vi "Data_base_server.vi"(0 "Raw Data Pathname":path, 1 "Results File Pathname":path, 3 "Clients time":dbl, 4 "Start time":dbl, 5 "End time":dbl, 6 "Average Meas Time (min)":dbl=100.0 format="%.1f", 7 "Channels from Client":string[][](array[string])=[["Data Base:Measurement:Type", "LDA & Cw"], ["Data Base:Position:No of Inst", "2"], ["Data Base:Position:X1", "-60"], ["Data Base:Position:X2", ""], ["Data Base:Position:Y1", "2"], ["Data Base:Position:Y2", "0.00"], ["Data Base:Position:Z1", "0.00"], ["Data Base:Position:Z2", "2.00"]], 8 "Average Sampling freq":sgl=100.0 format="%.1f", 9 "Rig Name":string) -> (14 "Channel names":string[](array[string])=["Data Base:DB:Filename", "Data Base:Start:Date", "Data Base:Start:Time", "EnFlo Tun:Job: Name", "EnFlo Tun:User: Name", "Data Base:Results:Folder", "Data Base:Results:Filename", "Data Base:Measurement:Type", "Data Base:X Axis:Max", "Data Base:X Axis:Min", "Data Base:Y Axis:Max", "Data Base:Y Axis:Min", "Data Base:Z Axis:Max", "Data Base:Z Axis:Min", "Data Base:No of:Measurements", "Data Base:Av Meas:Frequency (Hz)", "Data Base:Av Meas:Time (min)", "EnFlo Tun:labstrat1:Delta T", "EnFlo Tun:Heater Temp:Average", "EnFlo Tun:Inside:Velocity", "EnFlo Tun:Vorticity: Generators", "EnFlo Tun:Barrier Wall: Height", "EnFlo Tun:Roughness: Height", "EnFlo Tun:Side Wall: Separation", "EnFlo Tun:Obstacle/:Building", "EnFlo Tun:Obstacle: Orientation", "GMU:Source: Type", "GMU:Source: Height", "GMU:Release: Orientation", "GMU:Source:Meas Q", "GMU:Source:Meas Strength", "GMU:Trace: Gas", "GMU:Carrier: Gas", "GMU:Source:Release Temp", "GMU:Suction:Meas Q"], 15 "Channel values":string[](array[string])=["1999:May_1999:G3_3 HD_00006", "13/5/99", "1:55 pm", "National Power", "Paul Hayden", "BMT", "default", "LDA, Cw", "100.00", "-60.00", "2.00", "0.00", "0.00", "0.00", "10", "100.00", "100.00", "1.42", "26.63", "1.54", "\"7 quarter elipticals, 1 metre tall\"", "150mm", "20mm", "No sidewalls installed", "National Power Building", "30 deg", "D=17.5mm", "150 mm", "Vertical", "", "", "Ethane", "48% N2 in He", "", ""], 17 "spreadsheet string":string)   [LabVIEW 2022 SP3]
doc: "This is an example of using features of the VI Server as a client. It shows how you might browse from one or more applications that may be exporting data from one or more data stations. \n\nThe example shows how to query a server for its list of exported VIs, how to get references to the VIs, and how call them with the Call By Reference function."
uses:
  ADAM_Global.vi
  Sub VI's/Exp conditions/EnFlo_Tun_Setup_global.vi
  Anemometry/Anemometry Sub Vis/Globals/Constants_global.vi
panel:
  out "Output Array":string[][](array[string])
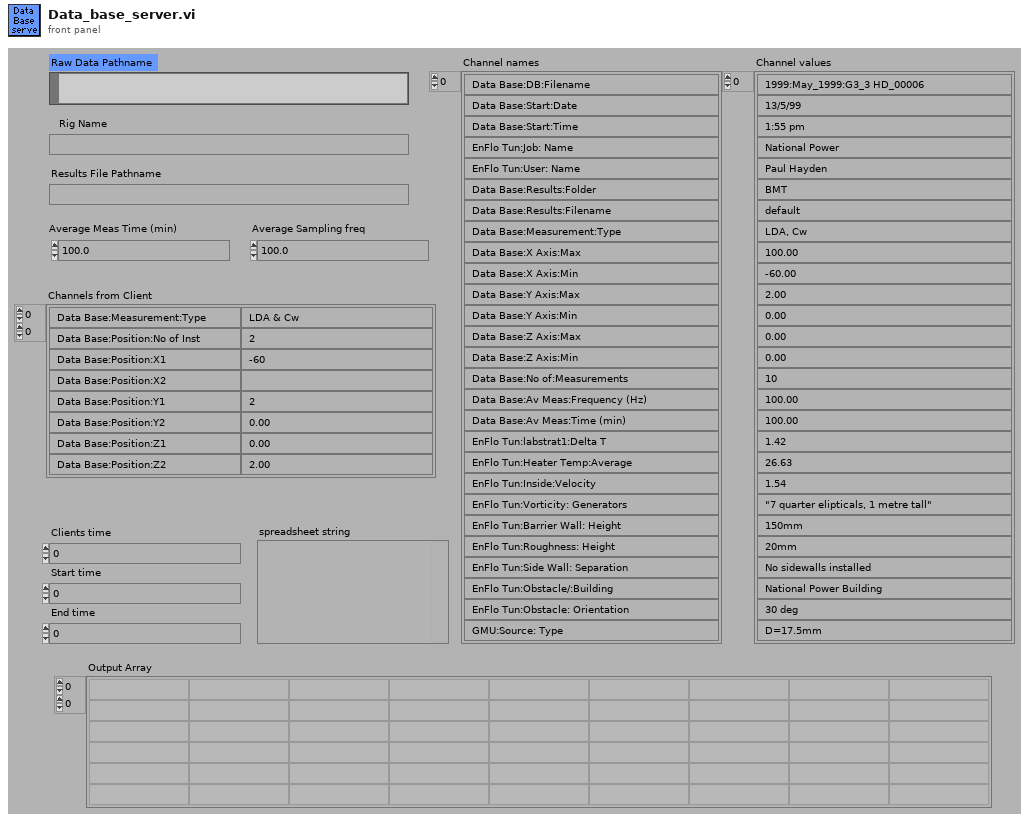
[diagram p1: front panel]
types:
  T1 = typedef "Ch_description_ADAM.ctl" = cluster{"Ch Name":string, "Type":T2, "Function":T3, "Ch State":T4, "Calibration type":T5, "A":dbl, "B":dbl, "C":dbl, "D":dbl, "Comments":string, "Address":T6, "String":string, "Duty":u16}
  T2 = typedef "Module_type_ADAM.ctl" = string
  T3 = typedef "Function_ADAM.ctl" = enum16{"Analogue Input", "Digital Input", "Event counter", "Event rate", "Analogue Output", "Digital Output", "Relay Output"}
  T4 = typedef "Channel_State.ctl" = enum16{"On", "Off", "Always On", "Always Off"}
  T5 = typedef "Calib_type_ADAM.ctl" = string
  T6 = typedef "Address.ctl" = cluster{"Main":i32, "Ch.":i32, "Sub":i32, "Port Name":string}
  T7 = cluster{"second":i32, "minute":i32, "hour":i32, "day of month":i32, "month":i32, "year":i32, "day of week":i32, "day of year":i32, "is DST":i32}
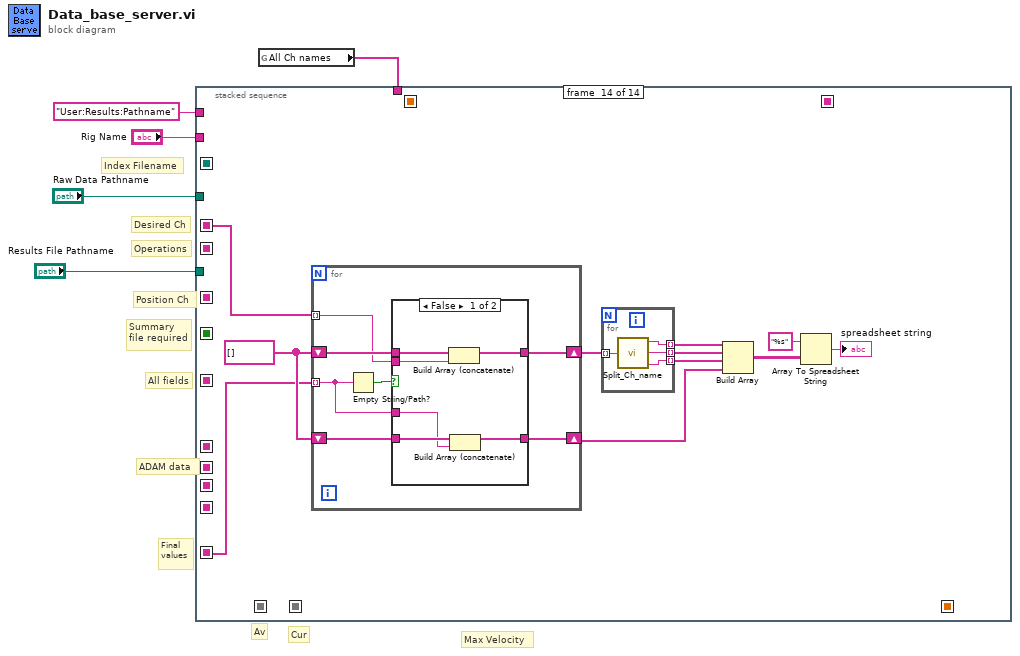
[diagram p0: block diagram]
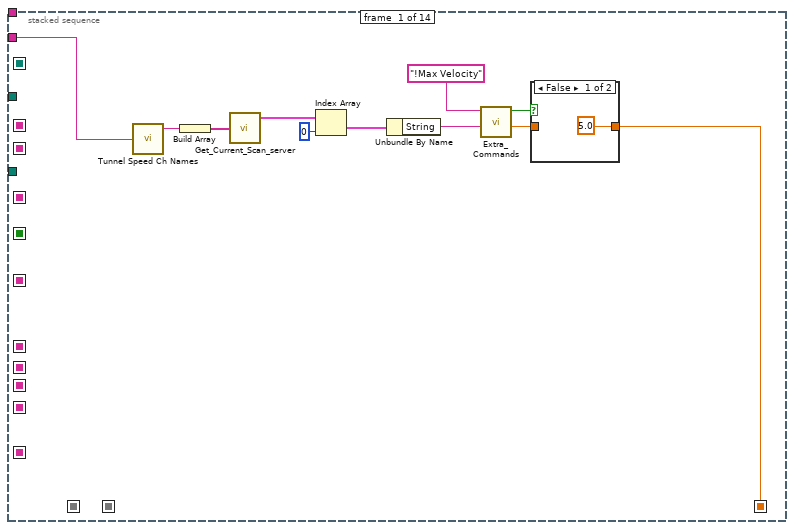
[diagram p2: hidden frame]
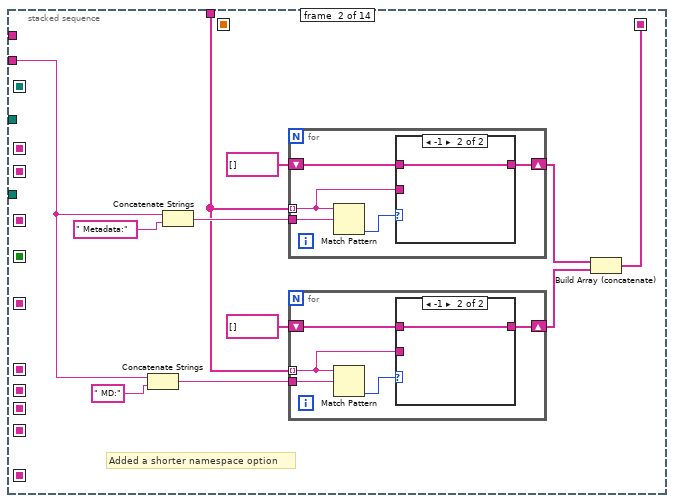
[diagram p4: hidden frame]
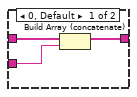
[diagram p5: hidden frame]
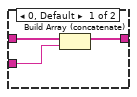
[diagram p6: hidden frame]
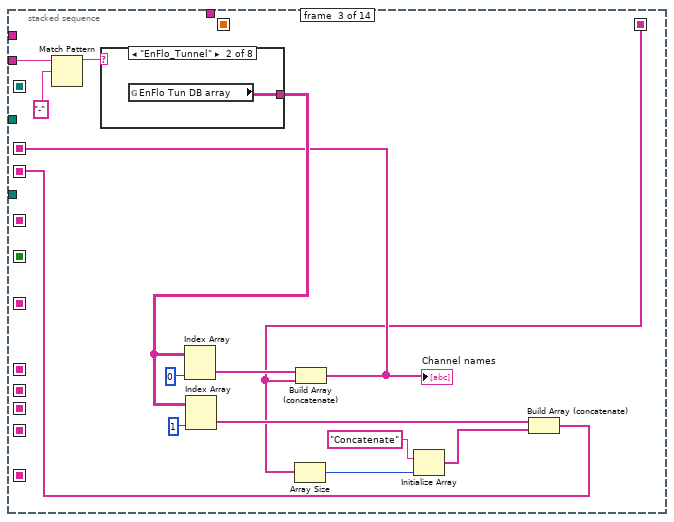
[diagram p7: hidden frame]
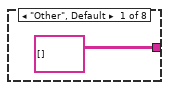
[diagram p8: hidden frame]
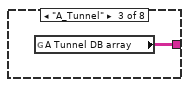
[diagram p9: hidden frame]
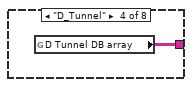
[diagram p10: hidden frame]
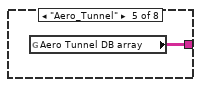
[diagram p11: hidden frame]
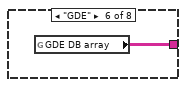
[diagram p12: hidden frame]
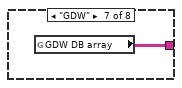
[diagram p13: hidden frame]
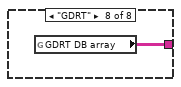
[diagram p14: hidden frame]
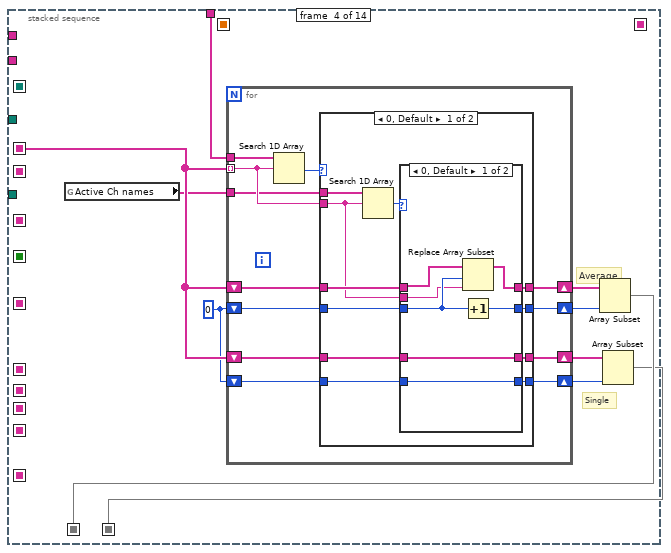
[diagram p15: hidden frame]
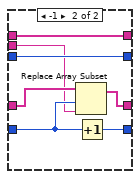
[diagram p16: hidden frame]
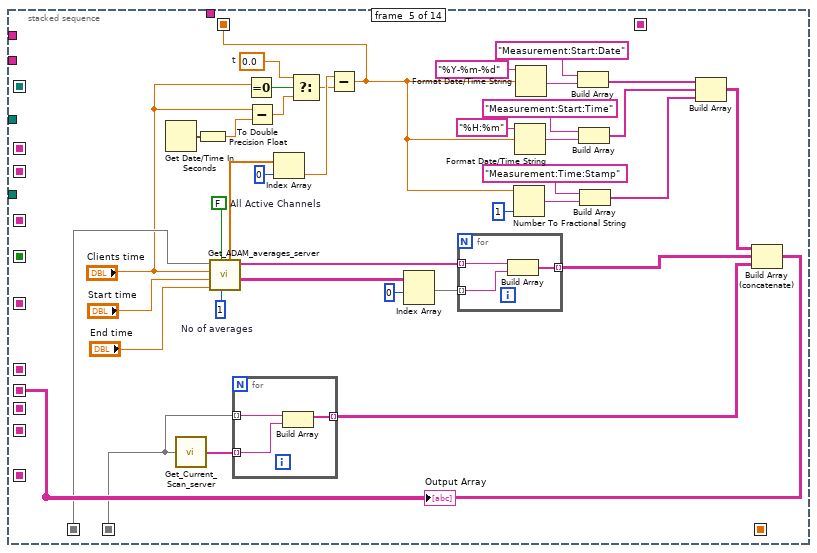
[diagram p18: hidden frame]
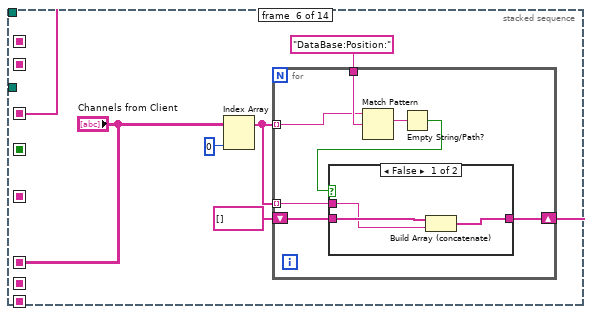
[diagram p19: hidden frame]
diagram:
  # "Max Velocity"
  # "Cur"
  # "Av"
  # "Index Filename"
  # "Desired Ch"
  # "Operations"
  # "Final\nvalues"
  # "Summary\nfile required"
  # "Position Ch"
  # "All fields"
  # "ADAM data"
  n1 = global read "ADAM_Global.vi" "All Ch names"() -> (w3:string[])
  n2 = stacked-sequence {
    seq-local: [_ _ w57 _ _ _ _ _ _ _ _ _ _ _] -> [_ _ _ w79 _ _ _ _ _ w218 _ _ w353 w363]
    seq-local: [_ _ _ _ w149 _ _ _ _ _ _ _ _ _] -> [_ _ _ _ _ _ _ _ w212 _ _ _ _ _]
    seq-local: [_ _ _ _ _ _ w199 _ _ _ _ _ _ _] -> [_ _ _ _ _ _ _ _ w211 _ _ _ _ _]
    seq-local: [_ _ _ _ _ _ _ _ w208 _ _ _ _ _] -> [_ _ _ _ _ _ _ _ _ w216 w318 _ _ _]
    seq-local: [_ _ _ _ _ _ _ w203 _ _ _ _ _ _] -> [_ _ _ _ _ _ _ _ w210 _ _ _ _ _]
    seq-local: [_ _ _ _ _ _ _ _ _ w220 _ _ _ _] -> [_ _ _ _ _ _ _ _ _ _ w324 _ w354 w362]
    seq-local: [_ _ _ _ _ w166 _ _ _ _ _ _ _ _] -> [_ _ _ _ _ _ _ w206 _ w217 _ _ _ _]
    seq-local: [_ _ _ _ _ "Channels from Client" _ _ _ _ _ _ _ _] -> [_ _ _ _ _ _ _ _ w209 w213 _ _ _ _]
    seq-local: [_ _ _ _ _ _ _ w204 _ _ _ _ _ _] -> [_ _ _ _ _ _ _ _ _ w219 _ _ _ _]
    seq-local: [_ _ w51 _ _ _ _ _ _ _ _ _ _ _] -> [_ _ _ _ _ _ _ _ _ w215 _ _ _ _]
    seq-local: [_ _ _ _ w123 _ _ _ _ _ _ _ _ _] -> [_ _ _ _ _ _ _ _ _ _ _ _ _ _]
    seq-local: [_ _ _ _ _ _ _ _ _ _ _ w341 _ _] -> [_ _ _ _ _ _ _ _ _ _ _ _ w351 _]
    seq-local: [_ _ _ w72 _ _ _ _ _ _ _ _ _ _] -> [_ _ _ _ w141 _ _ _ _ _ _ _ _ _]
    seq-local: [_ _ _ w71 _ _ _ _ _ _ _ _ _ _] -> [_ _ _ _ w140 _ _ _ _ _ _ _ _ _]
    seq-local: [_ w19 _ _ _ _ _ _ _ _ _ _ _ _] -> [_ _ w54 _ _ _ _ _ _ _ _ _ _ _]
    seq-local: [w7 _ _ _ _ _ _ _ _ _ _ _ _ _] -> [_ _ _ _ _ _ _ _ _ _ w311 _ _ _]
    tunnel: "User:Results:Pathname" -> [_ _ _ _ _ _ w187 _ _ _ _ _ w355 _]
    tunnel: "Results File Pathname" -> [_ _ _ _ _ _ w184 _ _ w214 _ _ _ _]
    tunnel: "Rig Name" -> [w16 w23 w50 _ _ _ _ _ _ _ w310 w348 _ _]
    tunnel: w3 -> [_ w24 _ w70 _ _ _ _ _ _ _ _ _ _]
    tunnel: "Raw Data Pathname" -> [_ _ _ _ _ _ _ w202 _ _ _ _ _ _]
    frame #0 {
      n3 = call "Tunnel Speed Ch Names.vi"("Rig Name"=w16) -> ("Dem Velocity"=w15:string)  [unwired: 2 in, 2 out]
      n4 = Build Array(w15) -> (w14:string[])
      n5 = call "Get_Current_Scan_server.vi"("Desired Channels"=w14) -> ("Ch Description Array"=w10:T1[])  [unwired: 2 out]
      n6 = Index Array(array=w10, index=0 ("Index")) -> (element=w13:T1)
      n7 = Unbundle By Name(w13) -> ("String"=w12:string)
      n8 = call "Extra_Commands.vi"("String to Search"=w12, "Command"="!Max Velocity") -> ("Numeric Value"=w6:dbl, "Command Found"=w8:bool)  [unwired: 1 in, 3 out]
      n9 = case shown="False" w8 {
        tunnel: [5.0 ("Max Velocity") w18] -> w7
        tunnel: w6 -> [_ w18]
        frame False {
        }
        frame True {
        }
      }
    }
    frame #1 {
      # "Added a shorter namespace option"
      n10 = Concatenate Strings(w23, " MD:" ("string")) -> (w25:string)
      n11 = Concatenate Strings(w23, " Metadata:") -> (w28:string)
      n12 = for {
        tunnel: w28 -> [w40]
        shift-right: [w41] -> w20
        shift-left: string[] [] -> [w42]
        tunnel: w24 -> [w39] mode=indexing
        n13 = Match Pattern(string=w39, regular expression=w40) -> (offset past match=w43:i32)  [unwired: 4 out]
        n14 = case shown="-1" w43 {
          tunnel: w42 -> [w46 w47]
          tunnel: [w44 w47] -> w41
          tunnel: w39 -> [w45 _]
          frame 0, Default {
            n15 = Build Array (concatenate)(w46, w45) -> (w44:string[])
          }
          frame -1 {
          }
        }
      }
      n16 = for {
        tunnel: w25 -> [w31]
        shift-right: [w32] -> w21
        shift-left: string[] [] -> [w33]
        tunnel: w24 -> [w30] mode=indexing
        n17 = Match Pattern(string=w30, regular expression=w31) -> (offset past match=w34:i32)  [unwired: 4 out]
        n18 = case shown="-1" w34 {
          tunnel: w33 -> [w37 w38]
          tunnel: [w35 w38] -> w32
          tunnel: w30 -> [w36 _]
          frame 0, Default {
            n19 = Build Array (concatenate)(w37, w36) -> (w35:string[])
          }
          frame -1 {
          }
        }
      }
      n20 = Build Array (concatenate)(w20, w21) -> (w19:string[])
    }
    frame #2 {
      n21 = Match Pattern(string=w50, regular expression="-") -> (before substring=w48:string)  [unwired: 1 in, 3 out]
      n22 = case shown="\"EnFlo_Tunnel\"" w48 {
        tunnel: [string[][] [] ("EnFlo Tun DB array") w63 w64 w65 w66 w67 w68 w69] -> w59
        frame "Other", Default {
        }
        frame "EnFlo_Tunnel" {
          n23 = global read "EnFlo_Tun_Setup_global.vi" "EnFlo Tun DB array"() -> (w63:string[][])
        }
        frame "A_Tunnel" {
          n24 = global read "EnFlo_Tun_Setup_global.vi" "A Tunnel DB array"() -> (w64:string[][])
        }
        frame "D_Tunnel" {
          n25 = global read "EnFlo_Tun_Setup_global.vi" "D Tunnel DB array"() -> (w65:string[][])
        }
        frame "Aero_Tunnel" {
          n26 = global read "EnFlo_Tun_Setup_global.vi" "Aero Tunnel DB array"() -> (w66:string[][])
        }
        frame "GDE" {
          n27 = global read "EnFlo_Tun_Setup_global.vi" "GDE DB array"() -> (w67:string[][])
        }
        frame "GDW" {
          n28 = global read "EnFlo_Tun_Setup_global.vi" "GDW DB array"() -> (w68:string[][])
        }
        frame "GDRT" {
          n29 = global read "EnFlo_Tun_Setup_global.vi" "GDRT DB array"() -> (w69:string[][])
        }
      }
      n30 = Index Array(array=w59, index (col)=0) -> (element=w58:string[])  [unwired: 1 in]
      n31 = Index Array(array=w59, index (col)=1) -> (element=w56:string[])  [unwired: 1 in]
      n32 = Array Size(array=w54) -> (size(s)=w55:i32)
      n33 = Build Array (concatenate)(w58, w54) -> (w57:string[])
      "Channel names" <- w57
      n34 = Initialize Array("Concatenate", w55) -> (w52:string[])
      n35 = Build Array (concatenate)(w56, w52) -> (w51:string[])
    }
    frame #3 {
      w77 = 0
      # "Single"
      # "Average"
      n36 = global read "ADAM_Global.vi" "Active Ch names"() -> (w78:string[])
      n37 = for {
        tunnel: w79 -> [w85] mode=indexing
        tunnel: w70 -> [w91]
        shift-right: [w89] -> w76
        shift-left: w79 -> [w88]
        shift-right: [w87] -> w74
        shift-left: w79 -> [w86]
        tunnel: w78 -> [w84]
        shift-right: [w80] -> w75
        shift-left: w77 -> [w81]
        shift-right: [w82] -> w73
        shift-left: w77 -> [w83]
        n38 = Search 1D Array(1D array=w91, element=w85) -> (index of element=w90:i32)  [unwired: 1 out]
        n39 = case shown="0, Default" w90 {
          tunnel: [w93 w120] -> w89
          tunnel: w88 -> [w94 w120]
          tunnel: [w99 w119] -> w87
          tunnel: w86 -> [w100 w119]
          tunnel: w85 -> [w92 _]
          tunnel: w84 -> [w102 _]
          tunnel: w83 -> [w98 w117]
          tunnel: [w97 w117] -> w82
          tunnel: w81 -> [w96 w118]
          tunnel: [w95 w118] -> w80
          frame 0, Default {
            n40 = Search 1D Array(1D array=w102, element=w92) -> (index of element=w101:i32)  [unwired: 1 out]
            n41 = case shown="0, Default" w101 {
              tunnel: w100 -> [w105 w116]
              tunnel: [w105 w115] -> w99
              tunnel: w98 -> [w104 w114]
              tunnel: [w104 w113] -> w97
              tunnel: w96 -> [w109 w112]
              tunnel: [w106 w112] -> w95
              tunnel: w94 -> [w108 w111]
              tunnel: [w107 w111] -> w93
              tunnel: w92 -> [w103 w110]
              frame 0, Default {
                n42 = Replace Array Subset(array=w108, new element=w103, index=w109) -> (w107:string[])
                n43 = Increment(x=w109) -> (x+1=w106:i32)
              }
              frame -1 {
                n44 = Replace Array Subset(array=w116, new element=w110, index=w114) -> (w115:string[])
                n45 = Increment(x=w114) -> (x+1=w113:i32)
              }
            }
          }
          frame -1 {
          }
        }
      }
      n46 = Array Subset(array=w76, length=w75) -> (w72:string[])  [unwired: 1 in]
      n47 = Array Subset(array=w74, length=w73) -> (w71:string[])  [unwired: 1 in]
    }
    frame #4 {
      w134 = 0.0  # t
      w142 = FALSE  # All Active Channels
      w158 = 1  # No of averages
      n48 = Get Date/Time In Seconds() -> (seconds since 1Jan1904=w130:timestamp)
      n49 = call "Get_Current_Scan_server.vi"("Desired Channels"=w140) -> ("String values"=w139:string[])  [unwired: 2 out]
      n50 = To Double Precision Float(number=w130) -> (double precision float=w137:dbl)
      n51 = call "Get_ADAM_averages_server.vi"("No of averages"=w158, "All Active Channels"=w142, "End time"="End time", "Start time"="Start time", "Clients time"="Clients time", "ADAM Ch Names"=w141) -> ("Values"=w145:string[][], "Titles"=w148:string[], "Times"=w156:dbl[])  [unwired: 2 out]
      n52 = for {
        tunnel: w139 -> [w161] mode=indexing
        tunnel: [w160] -> w138 mode=indexing
        tunnel: w140 -> [w159] mode=indexing
        n53 = Build Array(w159, w161) -> (w160:string[])
      }
      n54 = Equal To 0?(x="Clients time") -> (x = 0?=w135:bool)
      n55 = Subtract(x="Clients time", y=w137) -> (x-y=w136:dbl)
      n56 = Index Array(array=w156, index=0) -> (element=w132:dbl)
      n57 = Select(t=w134, s=w135, f=w136) -> (s? t:f=w131:dbl)
      n58 = Subtract(x=w132, y=w131) -> (x-y=w123:dbl)
      n59 = Index Array(array=w145, index (row)=0) -> (element=w147:string[])  [unwired: 1 in]
      n60 = for {
        tunnel: w148 -> [w164] mode=indexing
        tunnel: w147 -> [w163] mode=indexing
        tunnel: [w162] -> w150 mode=indexing
        n61 = Build Array(w164, w163) -> (w162:string[])
      }
      n62 = Number To Fractional String(number=w123, precision (6)=i16 1) -> (F-format string=w122:string)  [unwired: 2 in]
      n63 = Format Date/Time String(time format string (%c)="%H:%m", seconds (now)=w123) -> (date/time string=w126:string)  [unwired: 1 in]
      n64 = Format Date/Time String(time format string (%c)="%Y-%m-%d", seconds (now)=w123) -> (date/time string=w128:string)  [unwired: 1 in]
      n65 = Build Array("Measurement:Start:Date", w128) -> (w153:string[])
      n66 = Build Array("Measurement:Start:Time", w126) -> (w152:string[])
      n67 = Build Array("Measurement:Time:Stamp", w122) -> (w124:string[])
      n68 = Build Array(w153, w152, w124) -> (w151:string[][])
      n69 = Build Array (concatenate)(w151, w150, w138) -> (w149:string[][])
      "Output Array" <- w149
    }
    frame #5 {
      n70 = Index Array(array="Channels from Client", index (col)=0) -> (element=w168:string[])  [unwired: 1 in]
      n71 = for {
        tunnel: "DataBase:Position:" ("String to match") -> [w177]
        tunnel: w168 -> [w176] mode=indexing
        shift-right: [w171] -> w166
        shift-left: string[] [] -> [w172]
        tunnel: w168 -> [w173] mode=indexing
        n72 = Match Pattern(string=w176, regular expression=w177) -> (match substring=w175:string)  [unwired: 4 out]
        n73 = Empty String/Path?(string/path=w175) -> (empty?=w174:bool)
        n74 = case shown="False" w174 {
          tunnel: w173 -> [w178 _]
          tunnel: w172 -> [w180 w181]
          tunnel: [w179 w181] -> w171
          frame False {
            n75 = Build Array (concatenate)(w180, w178) -> (w179:string[])
          }
          frame True {
          }
        }
      }
    }
    frame #6 {
      n76 = Path To String(path=w184) -> (string=w186:string)
      n77 = Strip Path(path=w184) -> (name=w183:string)  [unwired: 1 out]
      n78 = Number To Fractional String(number="Average Meas Time (min)", precision (6)=i16 2) -> (F-format string=w196:string)  [unwired: 2 out]
      n79 = Number To Fractional String(number="Average Sampling freq", precision (6)=i16 2) -> (F-format string=w194:string)  [unwired: 2 out]
      n80 = Build Array("DataBase:Av Meas:Time (min)", w196) -> (w190:string[])
      n81 = Build Array("DataBase:Av Meas:Frequency (Hz)", w194) -> (w189:string[])
      n82 = Build Array("User:Results:Filename", w183) -> (w182:string[])
      n83 = Build Array(w187, w186) -> (w188:string[])
      n84 = Build Array(w188, w182, w190, w189) -> (w199:string[][])
    }
    frame #7 {
      n85 = Array Size(array=w206) -> (size(s)=w205:i32)
      n86 = Not Equal To 0?(x=w205) -> (x != 0?=w204:bool)
      n87 = Strip Path(path=w202) -> (stripped path=w201:path)  [unwired: 1 out]
      n88 = call "Path_2_String.vi"("Real Path"=w201) -> ("Path String"=w200:string)
      n89 = Build Array("DataBase:Raw_Data:Folder", w200) -> (w203:string[])
    }
    frame #8 {
      n90 = Build Array (concatenate)(w209, w212, w211, w210) -> (w208:string[][])
    }
    frame #9 {
      n91 = case shown="True" w219 {
        tunnel: [w222 w234] -> w220
        tunnel: w218 -> [w223 w233]
        tunnel: w217 -> [_ w232]
        tunnel: w216 -> [w224 w231]
        tunnel: w215 -> [_ w230]
        tunnel: w214 -> [_ w229]
        tunnel: w213 -> [_ w228]
        frame False {
          n92 = Index Array(array=w224, index (col)=1) -> (element=w225:string[])  [unwired: 1 in]
          n93 = Index Array(array=w224, index (col)=0) -> (element=w221:string[])  [unwired: 1 in]
          n94 = call "Merge_row_values.vi"("Present Row values"=w225, "Present Channels"=w221, "Desired Channels"=w223) -> ("Desired Row values"=w222:string[])  [unwired: 1 out]
        }
        frame True {
          # "Exists?"
          # "Ch names"
          # "Values"
          n95 = stacked-sequence {
            seq-local: [_ _ w265 _ _] -> [_ _ _ w281 w303]
            seq-local: [_ _ w261 _ _] -> [_ _ _ w285 w305]
            seq-local: [w242 _ _ _ _] -> [_ w248 w263 _ w306]
            seq-local: [_ w245 _ _ _] -> [_ _ w257 _ w304]
            seq-local: [_ _ w258 _ _] -> [_ _ _ _ w302]
            tunnel: [_ _ _ w286 _] -> w234
            tunnel: w233 -> [_ _ w264 w283 _]
            tunnel: w232 -> [_ _ w271 _ _]
            tunnel: w231 -> [_ _ w267 _ _]
            tunnel: w230 -> [_ _ _ w284 _]
            tunnel: w229 -> [w243 _ _ _ _]
            tunnel: w228 -> [_ w251 _ _ _]
            frame #0 {
              n96 = Strip Path(path=w243) -> (name=w236:string)  [unwired: 1 out]
              n97 = call "Add_filename_suffix.vi"("Filename"=w236) -> ("Base name"=w235:string)  [unwired: 1 in, 3 out]
              n98 = global read "Constants_global.vi" "Data Folder Local"() -> (w241:path)
              n99 = Concatenate Strings(w235, "_Sum.xls" ("Substring")) -> (w237:string)
              n100 = Build Array("Results_Summary_files", w237) -> (w240:string[])
              n101 = call "Build_Pathname.vi"("PathElements"=w240, "PathnameIn"=w241) -> ("AppendedPath"=w238:path)
              n102 = call "Create_directory_path.vi"("Path name"=w238) -> ("Path name Out"=w242:path)  [unwired: 2 in, 1 out]
            }
            frame #1 {
              n103 = Index Array(array=w251, index (col)=0) -> (element=w255:string[])  [unwired: 1 in]
              n104 = Search 1D Array(1D array=w255, element="Does the results file already exist?") -> (index of element=w252:i32)  [unwired: 1 out]
              n105 = Index Array(array=w251, index (row)=w252, index (col)=1 ("Index")) -> (element=w250:string)
              n106 = call "Does_file_exist_(simple).vi"("Pathname"=w248) -> ("exists?"=w246:bool)
              n107 = Not Equal?(x="FALSE", y=w250) -> (x != y?=w247:bool)
              n108 = And(x=w246, y=w247) -> (x .and. y?=w245:bool)
            }
            frame #2 {
              n109 = Build Array (concatenate)(w264, w271) -> (w270:string[])
              n110 = case shown="True" w257 {
                tunnel: w270 -> [w274 w280]
                tunnel: w263 -> [_ w279]
                tunnel: [w274 w278] -> w261
                tunnel: [string[][] [] ("Channel Values") w277] -> w259
                tunnel: [0 ("Offset from File End") w276] -> w258
                frame False {
                }
                frame True {
                  n111 = call "Read_Ch_data_file.vi"("Present Channels"=w280, "Output"=enum16{"All Ch data", "The last few rows"}."All Ch data", "Filename"=w279) -> ("Channel Values"=w277:string[][], "Merged Channels"=w278:string[], "Offset from File End"=w276:i64)  [unwired: 2 in, 2 out]
                }
              }
              n112 = Index Array(array=w267, index (col)=1) -> (element=w266:string[])  [unwired: 1 in]
              n113 = Index Array(array=w267, index (col)=0) -> (element=w262:string[])  [unwired: 1 in]
              n114 = call "Merge_row_values.vi"("Present Row values"=w266, "Present Channels"=w262, "Desired Channels"=w261) -> ("Desired Row values"=w260:string[])  [unwired: 1 out]
              n115 = Build Array (concatenate)(w259, w260) -> (w265:string[][])
            }
            frame #3 {
              n116 = call "Average_Column_Values.vi"("Present Values"=w281, "Present Channels"=w285, "Channel operations"=w284, "Channel names for operations"=w283) -> ("Desired Row values"=w282:string[])
              n117 = call "String_to_Pos_array.vi"("Channel values"=w281, "Channel names"=w285) -> ("Positions"=w289:dbl[][], "No of Inst"=w288:i32)
              n118 = while {
                tunnel: [w295] -> w287
                tunnel: w288 -> [w299]
                tunnel: w289 -> [w294]
                i -> [w292]
                stop <- w296 continue-if-true
                w290 = 3 ("x")
                n119 = Increment(x=w292) -> (x+1=w300:i32)
                n120 = Multiply(x=w290, y=w292) -> (x*y=w291:i32)
                n121 = Array Subset(array=w294, index (col)=w291, length (col)=w290) -> (w293:dbl[][])  [unwired: 2 in]
                n122 = call "Cal_Pos_Max_Min.vi"("Positions"=w293) -> ("Position Info"=w295:string[][], "Instrument moved?"=w297:bool)
                n123 = Less?(x=w300, y=w299) -> (x < y?=w298:bool)
                n124 = Compound Arithmetic op=AND(invert w297, w298) -> (w296:bool)
              }
              n125 = call "Replace_Channel_Values.vi"("Channels to replace"=w287, "Present Values"=w282, "Present Channels"=w283) -> ("Merged Row values"=w286:string[])  [unwired: 1 out]
            }
            frame #4 {
              w301 = TRUE  # Append last row only
              n126 = call "Write_Ch_data_file.vi"("Append last row only"=w301, "exists?"=w304, "Write offset fr file end"=w302, "Channel Values"=w303, "Channel names"=w305, "Filename"=w306) -> ()  [unwired: 2 in, 4 out]
            }
          }
        }
      }
    }
    frame #10 {
      n127 = Index Array(array=w318, index (col)=0) -> (element=w321:string[])  [unwired: 1 in]
      n128 = Concatenate Strings(w310, ":Pitot:Velocity" ("Substring")) -> (w323:string)
      n129 = Concatenate Strings(w310, ":Speed:Dem Velocity" ("Substring")) -> (w313:string)
      n130 = Concatenate Strings(w310, ":Speed:Calib Tweak" ("Substring")) -> (w312:string)
      n131 = Build Array(w313, w312, w323) -> (w320:string[])
      n132 = for {
        tunnel: w321 -> [w340]
        tunnel: w320 -> [w339] mode=indexing
        tunnel: [w338] -> w319 mode=indexing
        tunnel: [w337] -> w317 mode=indexing
        n133 = Search 1D Array(1D array=w340, element=w339) -> (index of element=w337:i32)  [unwired: 1 out]
        n134 = Greater Or Equal To 0?(x=w337) -> (x >= 0?=w338:bool)
      }
      n135 = call "Data_Base_logging.vi"("Rig Setup"=w310) -> ("Close Loop with Pitot?"=w308:bool)  [unwired: 3 out]
      n136 = And Array Elements(Boolean array=w319) -> (logical AND=w309:bool)
      n137 = And(x=w308, y=w309) -> (x .and. y?=w307:bool)
      n138 = case shown="True" w307 {
        tunnel: w318 -> [_ w331]
        tunnel: w317 -> [_ w329]
        tunnel: w310 -> [_ w327]
        tunnel: w311 -> [_ w325]
        frame False {
        }
        frame True {
          n139 = Index Array(array=w331, index (col)=1) -> (element=w330:string[])  [unwired: 1 in]
          n140 = for {
            tunnel: w330 -> [w336]
            tunnel: w329 -> [w335] mode=indexing
            tunnel: [w333] -> w328 mode=indexing
            n141 = Index Array(array=w336, index=w335) -> (element=w334:string)
            n142 = Fract/Exp String To Number(string=w334) -> (number=w333:dbl)  [unwired: 4 out]
          }
          n143 = call "Add_to_speed_calib_file.vi"("Max Velocity"=w325, "New Row"=w328, "Rig Name"=w327, "Mode"=enum16{"Add Row", "Get Error Value"}."Add Row") -> ()  [unwired: 2 in, 2 out]
        }
      }
      "Channel values" <- w324
    }
    frame #11 {
      n144 = Get Date/Time In Seconds() -> (seconds since 1Jan1904=w342:timestamp)
      n145 = call <vilib>:"LV70TimeStampToDateRec.vi"("time stamp"=w342) -> ("date time rec"=w350:T7)
      n146 = Unbundle By Name(w350) -> ("year"=w349:i32)
      n147 = Number To Decimal String(number=w349) -> (decimal integer string=w345:string)  [unwired: 1 out]
      n148 = Format Into String(format string="-%s.xls", initial string=w348, w345) -> (resulting string=w347:string)  [unwired: 1 in, 1 out]
      n149 = global read "Constants_global.vi" "Data Folder"() -> (w343:path)
      n150 = Build Array(w345, w348, w347) -> (w344:string[])
      n151 = call "Build_Pathname.vi"("PathElements"=w344, "PathnameIn"=w343) -> ("AppendedPath"=w341:path)
    }
    frame #12 {
      n152 = call "Update_Ch_data_file.vi"("Range"=enum16{"All Ch data", "The last few rows"}."The last few rows", "Channel to search on"=w355, "New Row values"=w354, "Present Channels"=w353, "Filename"=w351) -> ()  [unwired: 2 in, 5 out]
    }
    frame #13 {
      w364 = string[] []
      n153 = for {
        shift-right: [w373] -> w357
        shift-left: w364 -> [w374]
        shift-right: [w375] -> w361
        shift-left: w364 -> [w376]
        tunnel: w362 -> [w372] mode=indexing
        tunnel: w363 -> [w371] mode=indexing
        n154 = Empty String/Path?(string/path=w372) -> (empty?=w377:bool)
        n155 = case shown="False" w377 {
          tunnel: w376 -> [w383 w385]
          tunnel: [w382 w385] -> w375
          tunnel: w374 -> [w381 w384]
          tunnel: [w380 w384] -> w373
          tunnel: w372 -> [w379 _]
          tunnel: w371 -> [w378 _]
          frame False {
            n156 = Build Array (concatenate)(w383, w378) -> (w382:string[])
            n157 = Build Array (concatenate)(w381, w379) -> (w380:string[])
          }
          frame True {
          }
        }
      }
      n158 = for {
        tunnel: w361 -> [w370] mode=indexing
        tunnel: [w369] -> w360 mode=indexing
        tunnel: [w368] -> w359 mode=indexing
        tunnel: [w367] -> w358 mode=indexing
        n159 = call "Split_Ch_name.vi"("Ch name"=w370) -> ("Top level"=w369:string, "Middle"=w368:string, "Low level"=w367:string)
      }
      n160 = Build Array(w360, w359, w358, w357) -> (w356:string[][])
      n161 = Array To Spreadsheet String(array=w356, 3:"%s" ("format string")) -> (spreadsheet string=→"spreadsheet string":string)  [unwired: 1 out]
    }
  }
